vi "Post-Build Action - VxWorks.vi"(5 "Files Generated by Build":path[](array[path]), 6 "Top Level/Always Included VIs":path[](array[path]), 7 "Destination Path":path, 8 "error in (no error)":errorcluster, 9 "Target Name":string, 10 "Build Specification Name":string, 11 "Project Path":path) -> (0 "error out":errorcluster)   [LabVIEW 2016, in "Build VIs.lvlib"]
uses:
  Build VIs.lvlib
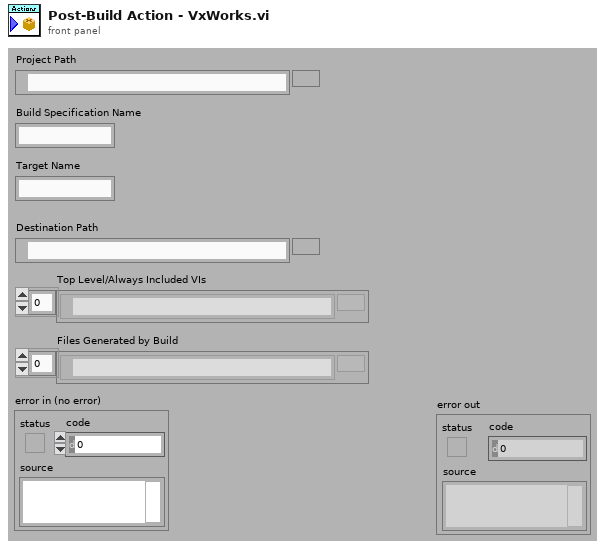
[diagram p1: front panel]
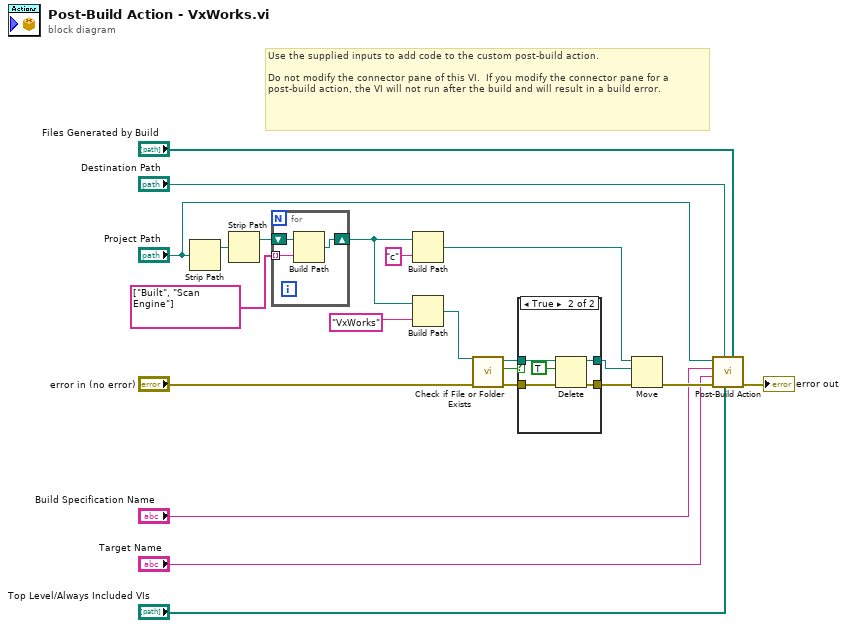
[diagram p0: block diagram]
diagram:
  # "Use the supplied inputs to add code to the custom post-build action.\n\nDo not modify the connector pane of this VI.  If you modify the connector pane for a post-build action, the VI will not run after the build and will result in a build error."
  n1 = Strip Path(path="Project Path") -> (stripped path=w22:path)  [unwired: 1 out]
  n2 = Strip Path(path=w22) -> (stripped path=w21:path)  [unwired: 1 out]
  n3 = for {
    shift-right: [w24] -> w19
    shift-left: w21 -> [w25]
    tunnel: string[] ["Built", "Scan Engine"] -> [w23] mode=indexing
    n4 = Build Path(base path=w25, name or relative path=w23) -> (appended path=w24:path)
  }
  n5 = Build Path(base path=w19, name or relative path="c") -> (appended path=w16:path)
  n6 = Build Path(base path=w19, name or relative path="VxWorks") -> (appended path=w3:path)
  n7 = call <vilib>:"Check if File or Folder Exists.vi"("error in (no error)"="error in (no error)", "path"=w3) -> ("error out"=w4:errorcluster, "file or folder exists?"=w1:bool, "dup path"=w2:path)  [unwired: 7 in]
  n8 = case shown="True" w1 {
    tunnel: [w26 w32] -> w15
    tunnel: [w27 w30] -> w14
    tunnel: w4 -> [w26 w29]
    tunnel: w2 -> [w27 w28]
    frame False {
    }
    frame True {
      n9 = Delete(path (use dialog)=w28, entire hierarchy (F)=TRUE, error in=w29) -> (deleted path=w30:path, error out=w32:errorcluster)  [unwired: 2 in, 1 out]
    }
  }
  n10 = Move(source path=w16, error in=w15, 10:w14) -> (error out=w13:errorcluster)  [unwired: 2 in, 2 out]
  n11 = call "Post-Build Action.vi"("Files Generated by Build"="Files Generated by Build", "Top Level/Always Included VIs"="Top Level/Always Included VIs", "Destination Path"="Destination Path", "error in (no error)"=w13, "Target Name"="Target Name", "Build Specification Name"="Build Specification Name", "Project Path"="Project Path") -> ("error out"=→"error out":errorcluster)  [unwired: 4 in]
